vi "Mode2-RAM.vi"() -> (3 "PAARD Super Mode":T4(array[cluster]))   [LabVIEW 2017]
uses:
  Classes/Sequence/SequenceSubvis/TestStep-StepType.ctl
  Classes/Sequence/SequenceSubvis/TestStepTypes.ctl
  Classes/Sequence/SequenceSubvis/RF Direction.ctl
  Classes/Sequence/SequenceSubvis/PolarizationSelect.ctl
  <vilib>/Utility/file.llb/Read Delimited Spreadsheet (DBL).vi
panel:
  in  "Polarization(s)":T1[](array[typedef])=[enum."Horizontal"]
  in  "Probe Vertical Polarization":bool
  in  "Probe Horizontal Polarization":bool
  in  "Play Button":bool
  in  "Pts":dbl
  in  "dPhi (deg)":dbl
  in  "Start Phi (deg)":dbl
  in  "Probe Tx/Rx":bool
  in  "Data File to Save":path
  in  "Upload TR Module file":path=path "C:/Users/Public/Documents/OU PAARD/mmWave_RF_Scanner/SupportFiles/example1.csv"
  out "# steps":i32
  out "length, bytes":i32 format="%.3p"
  in  "file path for testing":path
  in  "This is the File contents":cluster{"Z mm":dbl, "File Path":path}[](array[cluster])=[{"Z mm"=4.0, "File Path"=path ""}, {"Z mm"=0.0, "File Path"=path ""}, {"Z mm"=0.0, "File Path"=path ""}, {"Z mm"=0.0, "File Path"=path ""}, {"Z mm"=0.0, "File Path"=path ""}, {"Z mm"=0.0, "File Path"=path ""}, {"Z mm"=0.0, "File Path"=path ""}, {"Z mm"=0.0, "File Path"=path ""}, {"Z mm"=0.0, "File Path"=path ""}, {"Z mm"=0.0, "File Path"=path ""}, {"Z mm"=0.0, "File Path"=path ""}, {"Z mm"=0.0, "File Path"=path ""}, {"Z mm"=0.0, "File Path"=path ""}, {"Z mm"=0.0, "File Path"=path ""}, {"Z mm"=0.0, "File Path"=path ""}, {"Z mm"=0.0, "File Path"=path ""}, {"Z mm"=0.0, "File Path"=path ""}, {"Z mm"=0.0, "File Path"=path ""}, {"Z mm"=0.0, "File Path"=path ""}, {"Z mm"=0.0, "File Path"=path ""}, {"Z mm"=0.0, "File Path"=path ""}, {"Z mm"=0.0, "File Path"=path ""}, {"Z mm"=0.0, "File Path"=path ""}, {"Z mm"=0.0, "File Path"=path ""}, {"Z mm"=0.0, "File Path"=path ""}, {"Z mm"=0.0, "File Path"=path ""}, {"Z mm"=0.0, "File Path"=path ""}, {"Z mm"=0.0, "File Path"=path ""}, {"Z mm"=0.0, "File Path"=path ""}, {"Z mm"=0.0, "File Path"=path ""}, {"Z mm"=0.0, "File Path"=path ""}, {"Z mm"=0.0, "File Path"=path ""}, {"Z mm"=0.0, "File Path"=path ""}, {"Z mm"=0.0, "File Path"=path ""}, {"Z mm"=0.0, "File Path"=path ""}, {"Z mm"=0.0, "File Path"=path ""}, {"Z mm"=0.0, "File Path"=path ""}, {"Z mm"=0.0, "File Path"=path ""}, {"Z mm"=0.0, "File Path"=path ""}, {"Z mm"=0.0, "File Path"=path ""}, {"Z mm"=0.0, "File Path"=path ""}, {"Z mm"=0.0, "File Path"=path ""}, {"Z mm"=0.0, "File Path"=path ""}, {"Z mm"=0.0, "File Path"=path ""}, {"Z mm"=0.0, "File Path"=path ""}, {"Z mm"=0.0, "File Path"=path ""}, {"Z mm"=0.0, "File Path"=path ""}, {"Z mm"=0.0, "File Path"=path ""}, {"Z mm"=0.0, "File Path"=path ""}, {"Z mm"=0.0, "File Path"=path ""}, {"Z mm"=0.0, "File Path"=path ""}, {"Z mm"=0.0, "File Path"=path ""}, {"Z mm"=0.0, "File Path"=path ""}, {"Z mm"=0.0, "File Path"=path ""}, {"Z mm"=0.0, "File Path"=path ""}, {"Z mm"=0.0, "File Path"=path ""}, {"Z mm"=0.0, "File Path"=path ""}, {"Z mm"=0.0, "File Path"=path ""}, {"Z mm"=0.0, "File Path"=path ""}, {"Z mm"=0.0, "File Path"=path ""}, {"Z mm"=0.0, "File Path"=path ""}, {"Z mm"=0.0, "File Path"=path ""}, {"Z mm"=0.0, "File Path"=path ""}, {"Z mm"=0.0, "File Path"=path ""}, {"Z mm"=0.0, "File Path"=path ""}]
  in  "Antenna Tx/Rx":bool
  in  "H/V":bool
  in  "PAARD Mode 1":T5[](array[typedef])
  in  "UCAR Super Sequence":T5[](array[typedef])
  # "UI"
  # "Polarization = Probe Polarization"
  # "both H and V is ok.\n\nRule: only Tx or Rx is allowed."
  # "If there is a file, then\nignore the three numerics.\nElse if file is empty, generate FF positions from the three\nnumerics."
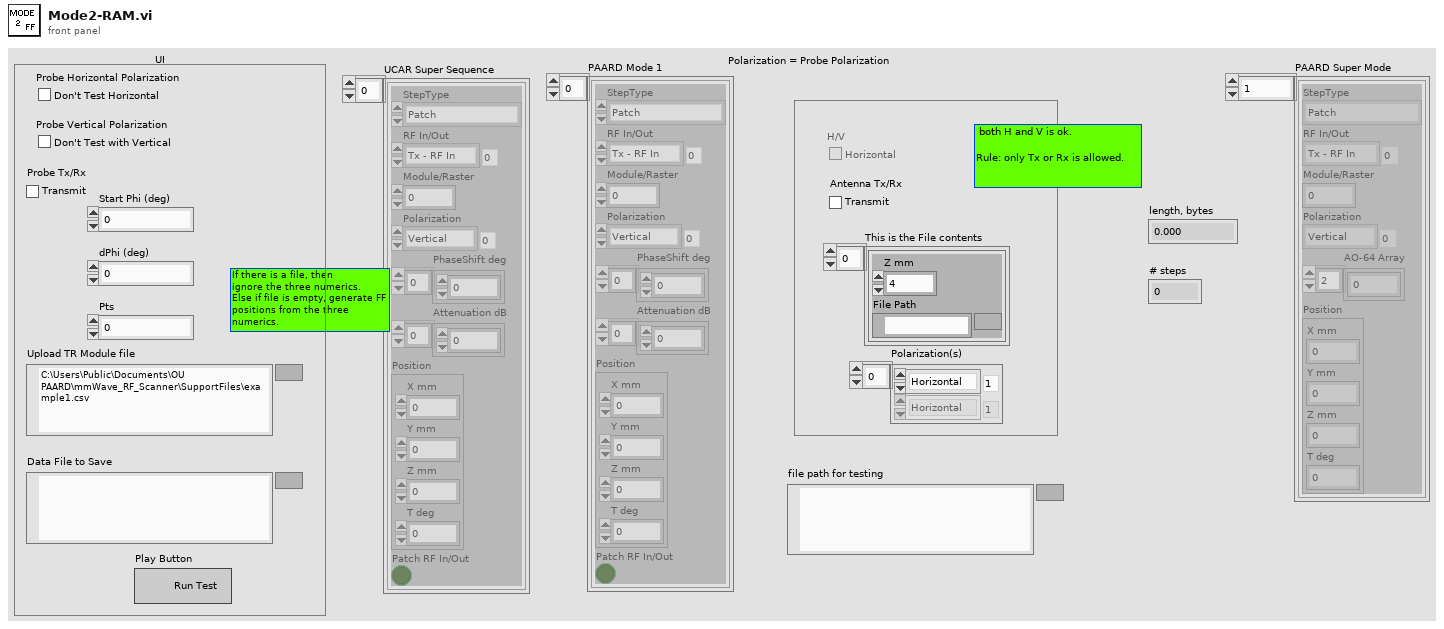
[diagram p1: front panel]
types:
  T1 = typedef "PolarizationSelect.ctl" = enum16{"Vertical", "Horizontal"}
  T2 = typedef "TestStepTypes.ctl" = enum16{"Patch", "Motion", "SweepTest", "RasterTest", "Finish", "64ModuleCfg"}
  T3 = typedef "RF Direction.ctl" = enum16{"Tx - RF In", "Rx - RF Out"}
  T4 = cluster{"StepType":T2, "RF In/Out":T3, "Module/Raster":i32, "Polarization":T1, "AO-64 Array":dbl[], "Position":cluster{"X mm":dbl, "Y mm":dbl, "Z mm":dbl, "T deg":dbl}}[]
  T5 = typedef "TestStep-StepType.ctl" = cluster{"StepType":T2, "RF In/Out":T3, "Module/Raster":i32, "Polarization":T1, "PhaseShift deg":dbl[], "Attenuation dB":dbl[], "Position":cluster{"X mm":dbl, "Y mm":dbl, "Z mm":dbl, "T deg":dbl}, "Patch RF In/Out":bool}
  T6 = cluster{"StepType":T2, "RF In/Out":T3, "Module/Raster":i32, "Polarization":T1, "AO-64 Array":dbl[], "Position":cluster{"X mm":dbl, "Y mm":dbl, "Z mm":dbl, "T deg":dbl}}
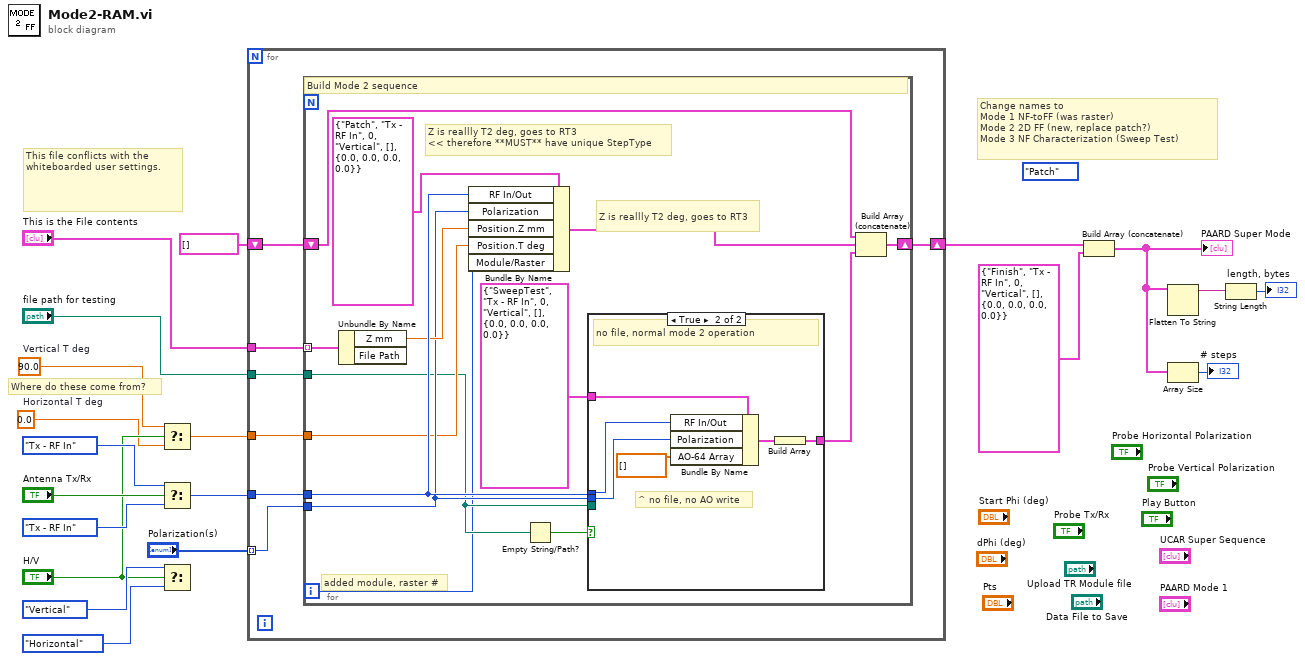
[diagram p0: block diagram]
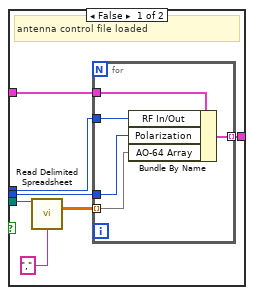
[diagram p2: hidden frame]
diagram:
  (unwired) TestStepTypes."Patch" ("StepType")
  w6 = 90.0  # Vertical T deg
  w5 = 0.0  # Horizontal T deg
  # "Change names to \nMode 1 NF-toFF (was raster) \nMode 2 2D FF (new, replace patch?)\nMode 3 NF Characterization (Sweep Test)"
  # "Where do these come from?"
  # "This file conflicts with the \nwhiteboarded user settings."
  n1 = Select(t=w6, s="H/V", f=w5) -> (s? t:f=w12:dbl)
  n2 = Select(t=RF_Direction."Tx - RF In" ("RF In/Out"), s="Antenna Tx/Rx", f=RF_Direction."Tx - RF In" ("RF In/Out")) -> (s? t:f=w15:T3)
  n3 = Select(t=PolarizationSelect."Vertical" ("Polarization"), s="H/V", f=PolarizationSelect."Horizontal" ("Polarization")) -> ()  [unwired: 1 out]
  n4 = for {
    tunnel: w15 -> [w27]
    tunnel: "This is the File contents" -> [w26]
    tunnel: w12 -> [w25]
    tunnel: "file path for testing" -> [w24]
    tunnel: "Polarization(s)" -> [w23] mode=indexing
    shift-right: [w21] -> w1
    shift-left: T4 [] -> [w22]
    n5 = for {
      tunnel: w27 -> [w39]
      tunnel: w23 -> [w35]
      tunnel: w26 -> [w38] mode=indexing
      shift-right: [w34] -> w21
      shift-left: w22 -> [w33]
      tunnel: w25 -> [w31]
      tunnel: w24 -> [w30]
      i -> [w28]
      # "Z is reallly T2 deg, goes to RT3\n<< therefore **MUST** have unique StepType"
      # "Z is reallly T2 deg, goes to RT3"
      # "added module, raster #"
      # "Build Mode 2 sequence"
      n6 = Unbundle By Name(w38) -> ("Z mm"=w37:dbl)  [unwired: 1 out]
      n7 = Bundle By Name(cluster=T6 {"StepType"=enum."Patch", "RF In/Out"=enum."Tx - RF In", "Module/Raster"=0, "Polarization"=enum."Vertical", "AO-64 Array"=[], "Position"={"X mm"=0.0, "Y mm"=0.0, "Z mm"=0.0, "T deg"=0.0}} ("Test"), "RF In/Out"=w39, "Polarization"=w35, "Position.Z mm"=w37, "Position.T deg"=w31, "Module/Raster"=w28) -> (w36:T6)
      n8 = Empty String/Path?(string/path=w30) -> (empty?=w29:bool)
      n9 = case shown="True" w29 {
        tunnel: T6 {"StepType"=enum."SweepTest", "RF In/Out"=enum."Tx - RF In", "Module/Raster"=0, "Polarization"=enum."Vertical", "AO-64 Array"=[], "Position"={"X mm"=0.0, "Y mm"=0.0, "Z mm"=0.0, "T deg"=0.0}} ("Test") -> [w48 w58]
        tunnel: w39 -> [w47 w56]
        tunnel: w35 -> [w45 w55]
        tunnel: [w44 w59] -> w32
        tunnel: w30 -> [w43 _]
        frame False {
          # "antenna control file loaded"
          n10 = call-poly <vilib>:"Read Delimited Spreadsheet.vi"("file path (dialog if empty)"=w43, "delimiter (\\t)"="," ("delimiter (\\t)")) -> ("all rows"=w46:dbl[][])  [unwired: 8 in, 5 out]
          n11 = for {
            tunnel: w48 -> [w53]
            tunnel: w47 -> [w52]
            tunnel: w46 -> [w51] mode=indexing
            tunnel: w45 -> [w50]
            tunnel: [w49] -> w44 mode=indexing
            n12 = Bundle By Name(cluster=w53, "RF In/Out"=w52, "Polarization"=w50, "AO-64 Array"=w51) -> (w49:T6)
          }
        }
        frame True {
          # "^ no file, no AO write"
          # "no file, normal mode 2 operation"
          n13 = Bundle By Name(cluster=w58, "RF In/Out"=w56, "Polarization"=w55, "AO-64 Array"=dbl[] []) -> (w57:T6)
          n14 = Build Array(w57) -> (w59:T4)
        }
      }
      n15 = Build Array (concatenate)(w33, w36, w32) -> (w34:T4)
    }
  }
  n16 = Build Array (concatenate)(w1, T6 {"StepType"=enum."Finish", "RF In/Out"=enum."Tx - RF In", "Module/Raster"=0, "Polarization"=enum."Vertical", "AO-64 Array"=[], "Position"={"X mm"=0.0, "Y mm"=0.0, "Z mm"=0.0, "T deg"=0.0}} ("Test")) -> (w8:T4)
  "PAARD Super Mode" <- w8
  n17 = Flatten To String(anything=w8) -> (data string=w10:string)  [unwired: 3 in, 2 out]
  n18 = Array Size(array=w8) -> (size(s)=→"# steps":i32)
  n19 = String Length(string=w10) -> (length=→"length, bytes":i32)
